vi "Deadband Joystick.vi"(1 "Deadband Amount":dbl=0.1 format="%#_13g", 2 "Joystick":string="Joystick") -> (0 "Deadbanded Axes":dbl[](array[numeric]))   [LabVIEW 2018]
uses:
  <vilib>/Rock Robotics/WPI/Utilities/WPI_GetSetVariantRefNum.vi
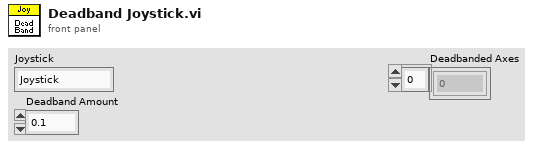
[diagram p1: front panel]
types:
  T1 = typedef "WPI_JoystickDevRef.ctl" = cluster{"Device":T2}
  T2 = typedef "WPI_JoystickDeviceEnum.ctl" = enum16{"USB 0", "USB 1", "USB 2", "USB 3", "USB 4", "USB 5"}
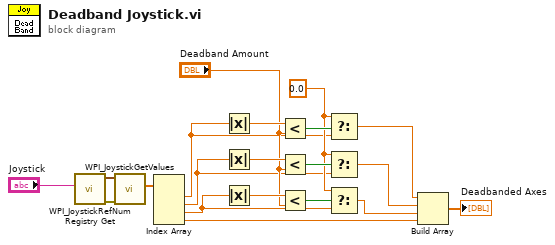
[diagram p0: block diagram]
diagram:
  w9 = 0.0
  n1 = call <vilib>:"WPI_JoystickRefNum Registry Get.vi"("refnum name"="Joystick") -> ("error out"=w19:errorcluster, "JoystickDevRef"=w18:T1)  [unwired: 9 in]
  n2 = call <vilib>:"WPI_JoystickGetValues.vi"("error in (no error)"=w19, "JoystickDevRef"=w18) -> ("Axes"=w17:dbl[])  [unwired: 5 in, 4 out]
  n3 = Index Array(array=w17) -> (element #1=w6:dbl, element #2=w7:dbl, element #3=w8:dbl, element #4=w2:dbl)  [unwired: 4 in]
  n4 = Absolute Value(x=w6) -> (abs(x)=w16:dbl)
  n5 = Absolute Value(x=w7) -> (abs(x)=w15:dbl)
  n6 = Absolute Value(x=w8) -> (abs(x)=w14:dbl)
  n7 = Less?(x=w16, y="Deadband Amount") -> (x < y?=w12:bool)
  n8 = Less?(x=w15, y="Deadband Amount") -> (x < y?=w11:bool)
  n9 = Less?(x=w14, y="Deadband Amount") -> (x < y?=w10:bool)
  n10 = Select(t=w9, s=w12, f=w6) -> (s? t:f=w5:dbl)
  n11 = Select(t=w9, s=w11, f=w7) -> (s? t:f=w4:dbl)
  n12 = Select(t=w9, s=w10, f=w8) -> (s? t:f=w3:dbl)
  n13 = Build Array(w5, w4, w3, w2) -> (→"Deadbanded Axes":dbl[])
